vi "Write_tcpClientQueue.vi"(8 "error in (no error)":errorcluster, 10 "tcpClientQueue":refnum<queue>, 11 "tcpServer in":refnum<class "TcpServer.lvclass">) -> (0 "error out":errorcluster, 3 "tcpServer out":refnum<class "TcpServer.lvclass">)   [LabVIEW 2018, in "TcpServer.lvclass"]
doc: "Create TCP client queue. This queue was created to send json packet to TCP Client."
uses:
  TcpServer.lvclass
  typedef/packetConnIDTypeDef.ctl
  TcpServer.lvclass/TcpServer.ctl
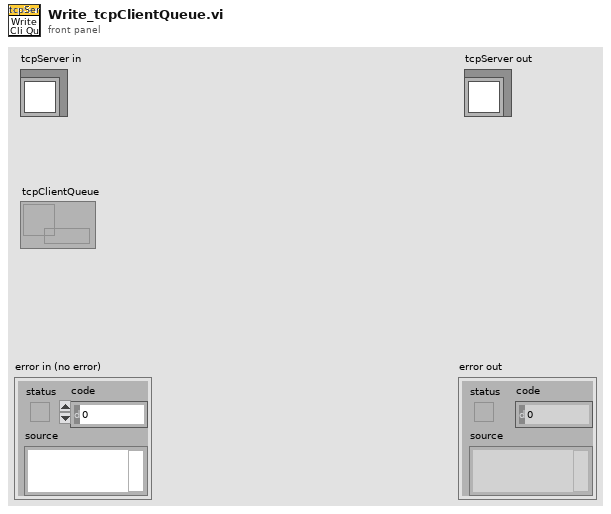
[diagram p1: front panel]
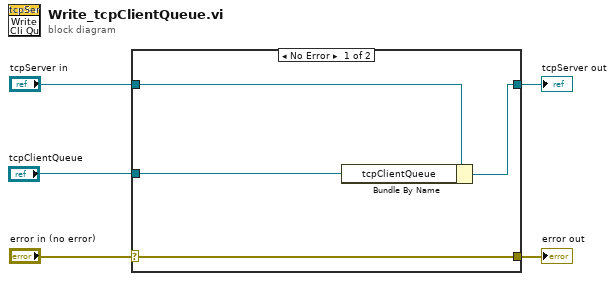
[diagram p0: block diagram]
diagram:
  n1 = case shown="No Error" "error in (no error)" {
    selector: "error in (no error)" -> [w9 w10]
    tunnel: [w9 w10] -> w4
    tunnel: [w7 w11] -> w2
    tunnel: "tcpServer in" -> [w8 w11]
    tunnel: "tcpClientQueue" -> [w6 _]
    frame No Error {
      n2 = Bundle By Name(cluster=w8, "tcpClientQueue"=w6) -> (w7:refnum<class "TcpServer.lvclass">)
    }
    frame Error {
    }
  }
  "error out" <- w4
  "tcpServer out" <- w2
